vi "Untitled 2 (SubVI).vi"   [LabVIEW 2020, in "Productos.lvlib"]
uses:
  Productos.lvlib
  <vilib>/Utility/sysdir.llb/System Directory Type.ctl
types:
  T1 = typedef "System Directory Type.ctl" = i32
  T2 = enum16{"open", "replace", "create", "open or create", "replace or create", "replace or create with confirmation"}
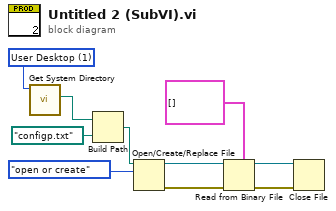
[diagram p0: block diagram]
diagram:
  w8 = T1 1 items=["User Home"=0, "User Desktop"=1, "User Documents"=2, "User Application Data"=3, "User Preferences"=4, "User Temporary"=5, "Public Documents"=6, "Public Application Data"=7, "Public Preferences"=8, "Public Cache"=13, "System Core Libraries"=9, "System Installed Libraries"=10, "Application Files"=11, "Boot Volume Root"=12] ("system directory type")
  n1 = call <vilib>:"Get System Directory.vi"("system directory type"=w8) -> ("system directory"=w7:path)  [unwired: 10 in]
  n2 = Build Path(base path=w7, name or relative path=path "configp.txt") -> (appended path=w5:path)
  n3 = Open/Create/Replace File(file path (use dialog)=w5, operation (0:open)=T2."open or create") -> (refnum out=w10:refnum<file>, error out=w4:errorcluster)  [unwired: 4 in, 1 out]
  n4 = Read from Binary File(5:cluster{"Numeric":dbl, "Boolean":bool}[] [] ("Array"), 8:w4, 11:w10) -> (0:w3:errorcluster, 3:w2:refnum<file>)  [unwired: 3 in, 2 out]
  n5 = Close File(refnum=w2, error in=w3) -> ()  [unwired: 2 out]
